vi "StrainMonitor.vi"() -> ()   [LabVIEW 2013]
panel:
  out "Warning":bool
  in  "?":bool
  out "Waveform Chart":i32[](graph)
  in  "Min Strain":i32=15
  in  "Max Strain":i32=30
  out "Ch16":i32
  out "Ch15":i32
  out "Ch14":i32
  out "Ch13":i32
  out "Ch12":i32
  out "Ch11":i32
  out "Ch10":i32
  out "Ch9":i32
  out "Ch8":i32
  out "Ch7":i32
  out "Ch6":i32
  out "Ch5":i32
  out "Ch4":i32
  out "Ch3":i32
  out "Ch2":i32
  out "Ch1":i32
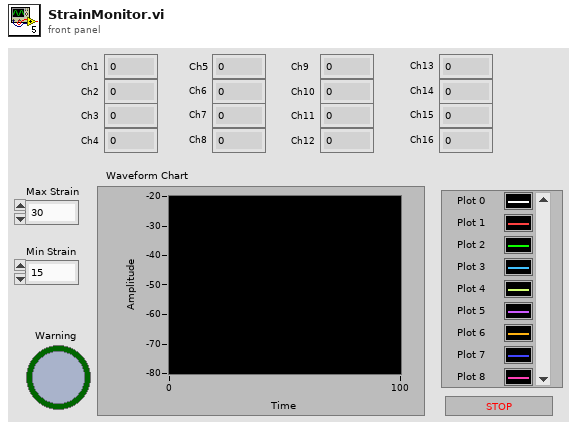
[diagram p1: front panel]
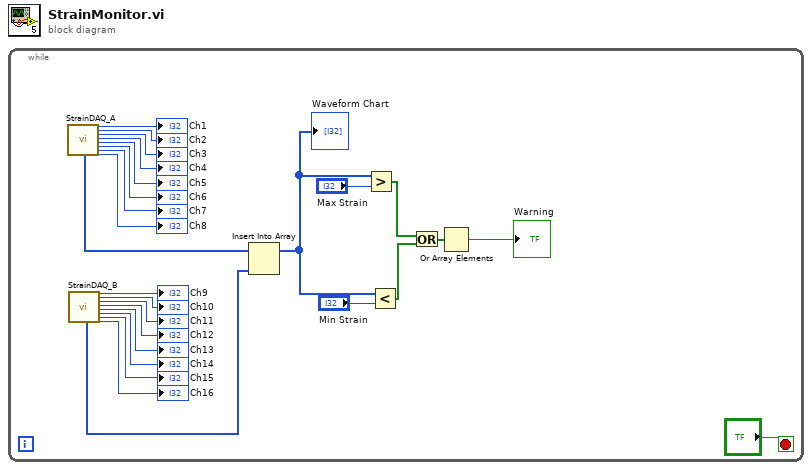
[diagram p0: block diagram]
diagram:
  n1 = while {
    stop <- "?" stop-if-true
    n2 = call "StrainDAQ_A.vi"() -> ("Strain Array"=w10:i32[], "element_1"=→"Ch1":i32, "element_2"=→"Ch2":i32, "element_3"=→"Ch3":i32, "element_4"=→"Ch4":i32, "element_5"=→"Ch5":i32, "element_6"=→"Ch6":i32, "element_7"=→"Ch7":i32, "element_8"=→"Ch8":i32)  [unwired: 19 in]
    n3 = call "StrainDAQ_B.vi"() -> ("Strain Array"=w9:i32[], "element_1"=→"Ch9":i32, "element_2"=→"Ch10":i32, "element_3"=→"Ch11":i32, "element_4"=→"Ch12":i32, "element_5"=→"Ch13":i32, "element_6"=→"Ch14":i32, "element_7"=→"Ch15":i32, "element_8"=→"Ch16":i32)  [unwired: 19 in]
    n4 = Insert Into Array(array=w10, new element=w9) -> (w2:i32[])  [unwired: 1 in]
    "Waveform Chart" <- w2
    n5 = Greater?(x=w2, y="Max Strain") -> (0:w6:bool[])
    n6 = Less?(x=w2, y="Min Strain") -> (x < y?=w5:bool[])
    n7 = Or(x=w6, y=w5) -> (x .or. y?=w4:bool[])
    n8 = Or Array Elements(Boolean array=w4) -> (logical OR=→"Warning":bool)
  }
